vi "Apertura File e Intestazioni.vi"() -> (0 "error out 2":errorcluster, 3 "Byte Stream File out":refnum<file>)   [LabVIEW 2018]
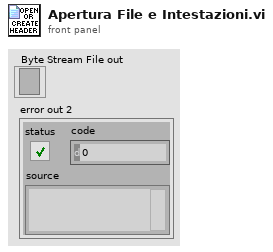
[diagram p1: front panel]
types:
  T1 = enum16{"open", "replace", "create", "open or create", "replace or create", "replace or create with confirmation"}
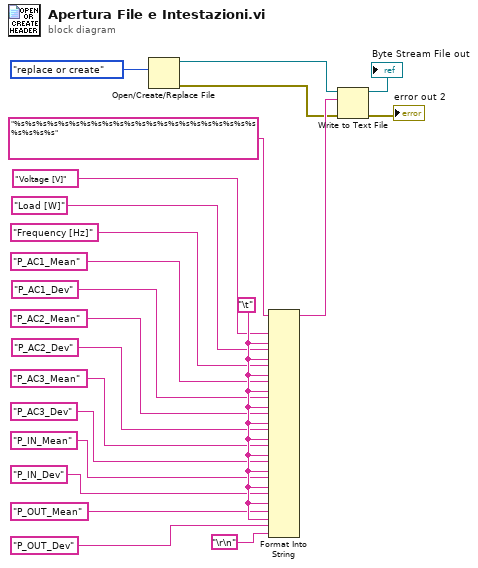
[diagram p0: block diagram]
diagram:
  w20 = "\t"
  n1 = Open/Create/Replace File(operation (0:open)=T1."replace or create") -> (refnum out=w11:refnum<file>, error out=w12:errorcluster)  [unwired: 5 in, 1 out]
  n2 = Format Into String(format string="%s%s%s%s%s%s%s%s%s%s%s%s%s%s%s%s%s%s%s%s%s%s%s%s%s%s", "Voltage [V]" ("input 1"), w20, "Load [W]" ("input 3"), w20, "Frequency [Hz]" ("input 3"), w20, "P_AC1_Mean" ("input 3"), w20, "P_AC1_Dev" ("input 3"), w20, "P_AC2_Mean" ("input 3"), w20, "P_AC2_Dev" ("input 3"), w20, "P_AC3_Mean" ("input 3"), w20, "P_AC3_Dev" ("input 3"), w20, "P_IN_Mean" ("input 3"), w20, "P_IN_Dev" ("input 3"), w20, "P_OUT_Mean" ("input 3"), w20, "P_OUT_Dev" ("input 3"), "\r\n") -> (resulting string=w13:string)  [unwired: 2 in, 1 out]
  n3 = Write to Text File(file (use dialog)=w11, text=w13, error in=w12) -> (refnum out=→"Byte Stream File out":refnum<file>, error out=→"error out 2":errorcluster)  [unwired: 1 in, 1 out]
